vi "Add RUN Window.vi"(6 "Index":i32=-1, 8 "error in (no error)":errorcluster, 9 "Schedule Block":refnum<class "Schedule Block.lvclass">, 10 "Modify":bool, 11 "Scheduler in":refnum<class "Scheduler.lvclass">=refnum) -> (0 "error out":errorcluster={"status"=TRUE, "code"=5666, "source"="desktop-pk571s1: Scheduler: Scheduler::Error while updating subpanels in the Add Run"}, 3 "Scheduler out":refnum<class "Scheduler.lvclass">)   [LabVIEW 2020, in "CIRCUS_uServices.lvlib" / "Scheduler.lvlib"]
uses:
  Scheduler.lvlib
  Run Utilities/Scan SBlock/Scan Mode Panel.vi
  Run Utilities/Scan SBlock/Scan SBlock.lvclass
  Scheduler Consumer Case Selector.ctl
  Scheduler.lvclass
  Add RUN Output Data Packet.ctl
  TALOS/TALOS_PPL.lvlibp
  TALOS/TALOS_PPL.lvlibp/Father of all uServices/Father of all uServices/Father of all uServices.lvclass
  TALOS/TALOS_PPL.lvlibp/Support VIs/Global Memory.vi
  TALOS/TALOS_PPL.lvlibp/Interfaces/FPGA Interface/FPGA Interface.lvclass
  Run Utilities/Schedule Block/Schedule Block.lvclass
  C:/Users/marco/Documents/GitHub_Lab/CIRCUS/TALOS/TALOS_PPL.lvlibp/Father of all uServices/Father of all uServices/Father of all uServices.lvclass
  C:/Users/marco/Documents/GitHub_Lab/CIRCUS/TALOS/TALOS_PPL.lvlibp/Ancestor/Ancestor/Ancestor.lvclass
  C:/Users/marco/Documents/GitHub_Lab/CIRCUS/TALOS/Actor Framework.lvlibp/1abvi3w/vi.lib/ActorFramework/Actor/Actor.lvclass
  C:/Users/marco/Documents/GitHub_Lab/CIRCUS/CIRCUS uServices et al/Scheduler/Scheduler.lvclass
  Run Utilities/Scan SBlock/Parameter name with value - GUI.ctl
  TALOS/Actor Framework.lvlibp/1abvi3w/vi.lib/ActorFramework/Message Enqueuer/Message Enqueuer.lvclass
  TALOS/Actor Framework.lvlibp/1abvi3w/vi.lib/ActorFramework/Message Priority Queue/Message Priority Queue.lvclass
  Classes/Log/Log.lvclass
  Classes/Config/Config.lvclass
panel:
  in  "Subpanels Map":map{string, refnum<vi>}(c390)={"Optimiser"=refnum, "Scan"=refnum}
  in  "Parameters Map":map{string, string[]}(c390)
  in  "FPGA Selector":string(combo)
  in  "Obsv to check":string[](array[string]) caption="Quality of Run Check"
  in  "Mode":string(combo)="Scan"
  in  "Common Parameters":T1[](array[typedef])
  in  "Cancel":bool
  in  "OK":bool
  in  "Number of repetitions":u16=1 min=1
  in  "Browse":bool
  in  "Script Path":path
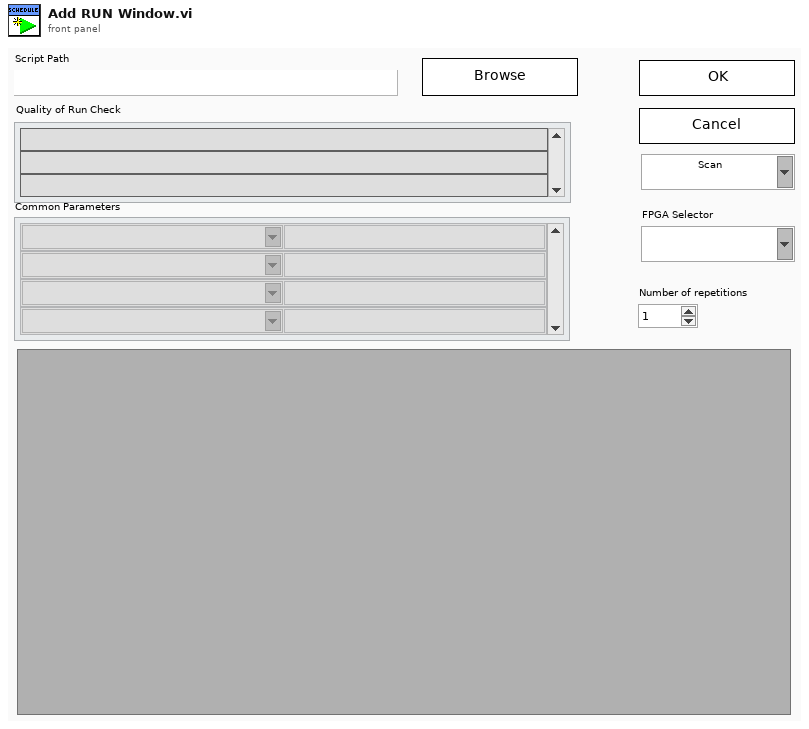
[diagram p1: front panel]
types:
  T1 = typedef "CIRCUS_uServices.lvlib/Run Utilities.lvlib/Scan SBlock.lvclass/Parameter name with value - GUI.ctl" = cluster{"Parameter Name":string, "Parameter Value":string}
  T2 = typedef "CIRCUS_uServices.lvlib/Scheduler.lvlib/Scheduler.lvclass/Add RUN Output Data Packet.ctl" = cluster{"Index":i32, "Schedule Block":refnum<class "Schedule Block.lvclass">}
  T3 = typedef "CIRCUS_uServices.lvlib/Scheduler.lvlib/Scheduler.lvclass/Scheduler Consumer Case Selector.ctl" = enum16{"Add SBlock", "Update GUI", "Move SBlock", "Select SBlock", "Update Cont.", "Load", "Save", "Reset", "Send to Tamer", "Edit SBlock", "Duplicate SBlock", "Delete SBlock", "Update SBlock", "Init", "Split/Combine Schedules", "Reschedule", "Load Parameters"}
  T4 = cluster{"result string":string, "String":string, "result string":string}[]
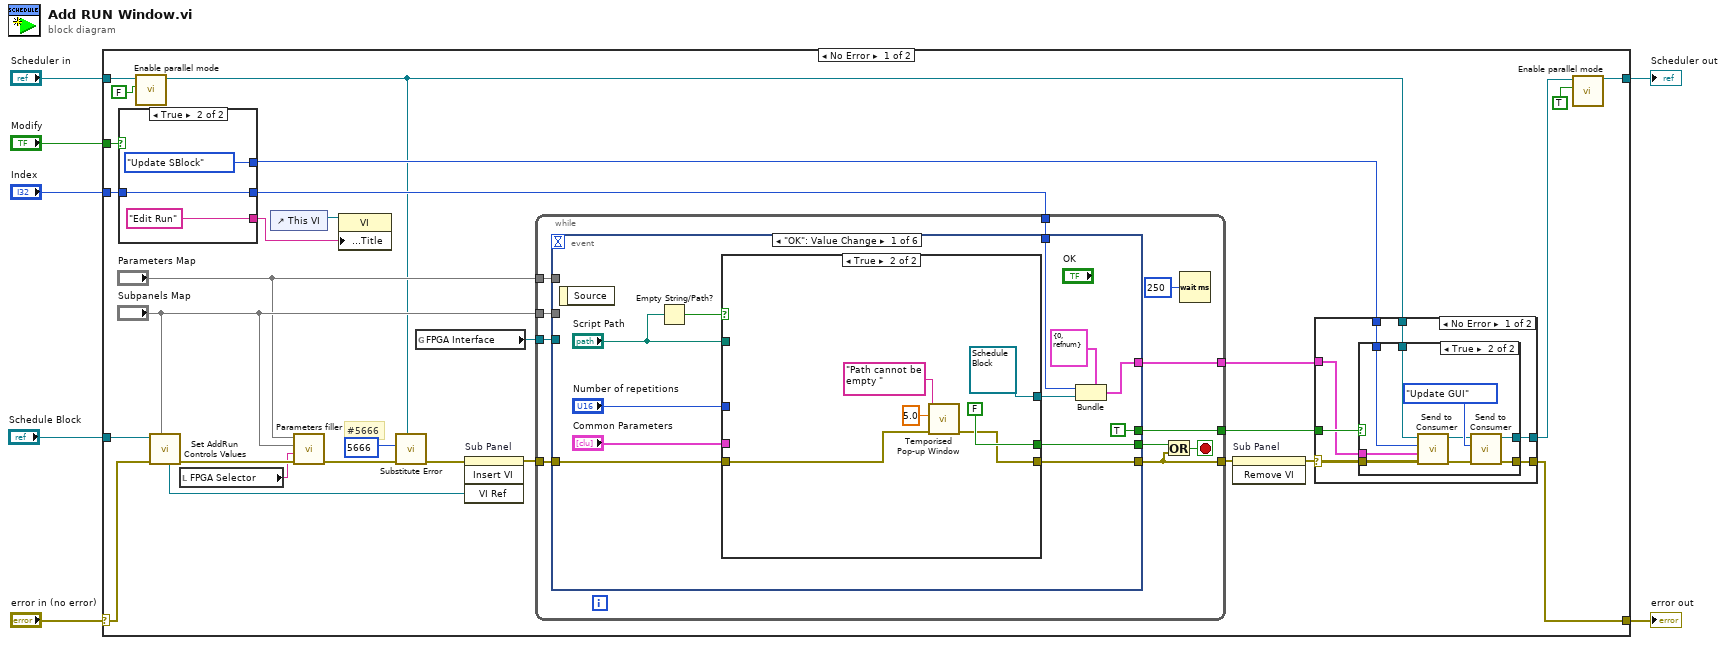
[diagram p0: block diagram]
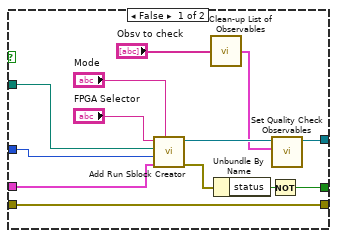
[diagram p2: hidden frame]
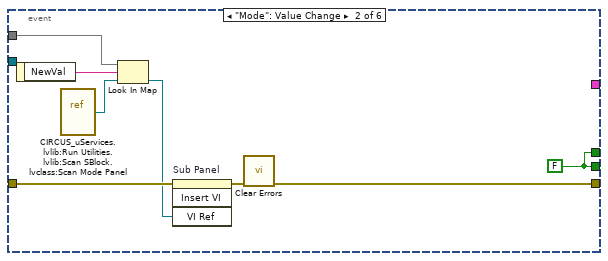
[diagram p3: hidden frame]
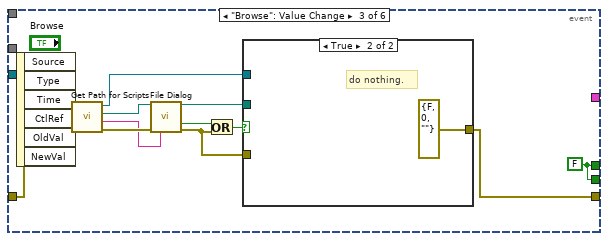
[diagram p4: hidden frame]
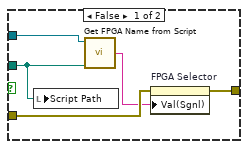
[diagram p5: hidden frame]
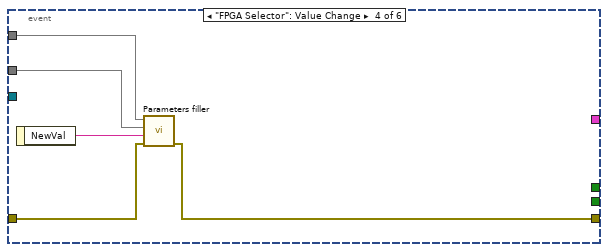
[diagram p6: hidden frame]
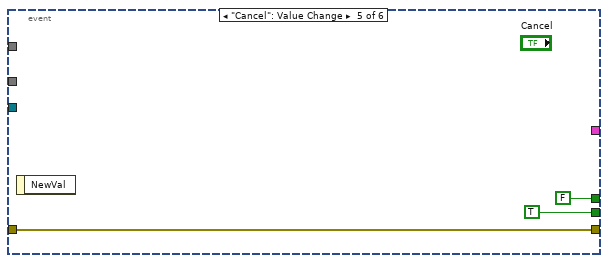
[diagram p7: hidden frame]
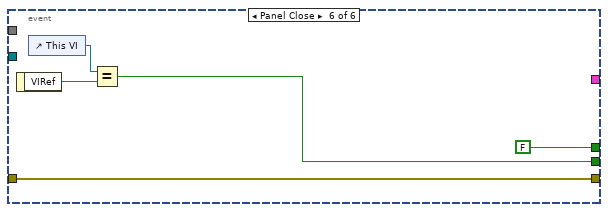
[diagram p8: hidden frame]
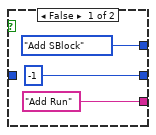
[diagram p11: hidden frame]
diagram:
  n1 = case shown="No Error" "error in (no error)" {
    selector: "error in (no error)" -> [w13 w145]
    tunnel: [w23 w145] -> w4
    tunnel: [w22 w144] -> w5
    tunnel: "Scheduler in" -> [w28 w144]
    tunnel: "Modify" -> [w34 _]
    tunnel: "Schedule Block" -> [w15 _]
    tunnel: "Index" -> [w30 _]
    frame No Error {
      # "#5666"
      n2 = case shown="True" w34 {
        tunnel: [Scheduler_Consumer_Case_Selector."Add SBlock" ("Shifter Panel Consumer Case Selector") Scheduler_Consumer_Case_Selector."Update SBlock" ("Shifter Panel Consumer Case Selector")] -> w32
        tunnel: w30 -> [_ w142]
        tunnel: [-1 ("Index") w142] -> w29
        tunnel: ["Add Run" ("Front Panel Window:Title") "Edit Run" ("Front Panel Window:Title")] -> w19
        frame False {
        }
        frame True {
        }
      }
      n3 = call-dynamic "Enable parallel mode.vi"("Enable"=FALSE, "Scheduler in"=w28) -> ("Scheduler out"=w10:refnum<class "Scheduler.lvclass">)  [unwired: 8 in, 1 out]
      n4 = call "Set AddRun Controls Values.vi"("Subpanels Map"="Subpanels Map", "error in"=w13, "Schedule Block"=w15) -> ("error out"=w16:errorcluster, "SubPanel VI out"=w9:refnum<vi>)  [unwired: 6 in, 1 out]
      n5 = local read "FPGA Selector"() -> (w11:string)
      n6 = control-ref of="This VI"() -> (w18:refnum<vi>)
      n7 = call "Parameters filler.vi"("error in (no error)"=w16, "FPGA Name"=w11, "Subpanels Map"="Subpanels Map", "Parameters Map"="Parameters Map") -> ("error out"=w12:errorcluster)  [unwired: 7 in]
      n8 = property class="VI"(reference=w18, "Front Panel.Title"=w19) -> ()  [unwired: 1 in, 2 out]
      n9 = call "Substitute Error.vi"("LabVIEW Object"=w10, "error in (no error)"=w12, "Error Code"=5666) -> ("error out"=w26:errorcluster)  [unwired: 8 in]
      n10 = global read "Global Memory.vi" "FPGA Interface"() -> (w20:refnum<class "FPGA Interface.lvclass">)
      n11 = invoke on="Sub Panel" class="SubPnl" method="Insert VI"(error in=w26, "VI Ref"=w9) -> (error out=w8:errorcluster)  [unwired: 2 in, 3 out]
      n12 = while {
        tunnel: [w37] -> w35
        tunnel: w8 -> [w47]
        tunnel: [w44] -> w33
        tunnel: [w43] -> w31
        tunnel: w29 -> [w42]
        tunnel: w20 -> [w41]
        tunnel: "Subpanels Map" -> [w40]
        tunnel: "Parameters Map" -> [w39]
        stop <- w46 stop-if-true
        n13 = event shown="[0] \"OK\": Value Change" {
          selector: _ -> [_ _ _ _ _ _]
          dyn-events: _ -> [_ _ _ _ _ _]
          timeout: _ -> [_ _ _ _ _ _]
          tunnel: [w55 w79 w97 _ TRUE w114] -> w38
          tunnel: [w48 w81 w98 w105 w111 w117] -> w37
          tunnel: w47 -> [w56 w82 w91 w106 w111 w117]
          tunnel: [w52 _ _ _ _ _] -> w44
          tunnel: [TRUE w79 w97 _ FALSE FALSE] -> w43
          tunnel: w42 -> [w50 _ _ _ _ _]
          tunnel: w41 -> [_ _ w92 _ _ _]
          tunnel: w40 -> [_ w83 _ w107 _ _]
          tunnel: w39 -> [_ _ _ w108 _ _]
          event "OK": Value Change {
            n14 = event-data() -> ()  [unwired: 1 in, 1 out]
            n15 = Empty String/Path?(string/path="Script Path") -> (empty?=w57:bool)
            n16 = case shown="True" w57 {
              tunnel: "Number of repetitions" -> [w63 _]
              tunnel: "Script Path" -> [w67 _]
              tunnel: w56 -> [w70 w78]
              tunnel: [w72 FALSE] -> w55
              tunnel: [w69 refnum<class "Schedule Block.lvclass"> refnum ("Schedule Block out")] -> w51
              tunnel: "Common Parameters" -> [w66 _]
              tunnel: [w70 w73] -> w48
              frame False {
                n17 = call "Add Run Sblock Creator.vi"("SBlock type"="Mode", "Common Parameters"=w66, "Number of repetitions"=w63, "Script Path"=w67, "FPGA Name"="FPGA Selector") -> ("error out"=w65:errorcluster, "Schedule Block out"=w64:refnum<class "Schedule Block.lvclass">)  [unwired: 5 in]
                n18 = call "Clean-up List of Observables.vi"("Obsv to check"="Obsv to check") -> ("Array"=w60:T4)
                n19 = Unbundle By Name(w65) -> ("status"=w71:bool)
                n20 = Not(x=w71) -> (.not. x?=w72:bool)
                n21 = call-dynamic "Set Quality Check Observables.vi"("Obsv to check"=w60, "Schedule Block in"=w64) -> ("Schedule Block out"=w69:refnum<class "Schedule Block.lvclass">)  [unwired: 8 in, 1 out]
              }
              frame True {
                n22 = call "Temporised Pop-up Window.vi"("error in (no error)"=w78, "Timeout"=5.0, "Text"="Path cannot be empty ") -> ("error out"=w73:errorcluster)  [unwired: 8 in]
              }
            }
            n23 = Bundle(cluster=T2 {"Index"=0, "Schedule Block"=refnum} ("Cluster"), "Index"=w50, "Schedule Block"=w51) -> (w52:T2)
          }
          event "Mode": Value Change {
            w79 = FALSE
            n24 = event-data() -> ("NewVal"=w85:string)  [unwired: 1 in]
            n25 = vi-ref "CIRCUS_uServices.lvlib:Run Utilities.lvlib:Scan SBlock.lvclass:Scan Mode Panel.vi"() -> (w84:refnum<vi>)
            n26 = Look In Map(map=w83, key=w85, default value=w84) -> (value=w80:refnum<vi>)  [unwired: 1 out]
            n27 = invoke on="Sub Panel" class="SubPnl" method="Insert VI"(error in=w82, "VI Ref"=w80) -> (error out=w86:errorcluster)  [unwired: 2 in, 3 out]
            n28 = call <vilib>:"Clear Errors.vi"("error in (no error)"=w86) -> ("error out"=w81:errorcluster)  [unwired: 5 in, 1 out]
          }
          event "Browse": Value Change {
            w97 = FALSE
            n29 = event-data() -> ()  [unwired: 1 in, 6 out]
            n30 = call-dynamic "Get Path for Scripts.vi"("error in (no error)"=w91, "FPGA Interface in"=w92) -> ("error out"=w90:errorcluster, "File pattern"=w89:string, "Path"=w88:path, "FPGA Interface out"=w87:refnum<class "FPGA Interface.lvclass">)  [unwired: 6 in]
            n31 = call "File Dialog"("start path"=w88, "error in"=w90, "pattern (all files)"=w89) -> ("selected path"=w94:path, "cancelled"=w96:bool, "error out"=w93:errorcluster)  [unwired: 9 in, 1 out]
            n32 = Or(x=w96, y=w93) -> (x .or. y?=w95:bool)
            n33 = case shown="True" w95 {
              tunnel: w94 -> [w103 _]
              tunnel: [w101 errorcluster {"status"=FALSE, "code"=0, "source"=""} ("error out")] -> w98
              tunnel: w93 -> [w100 _]
              tunnel: w87 -> [w102 _]
              frame False {
                n34 = local write "Script Path"(w103) -> ()
                n35 = call-dynamic "Get FPGA Name from Script.vi"("file"=w103, "FPGA Interface"=w102) -> ("FPGA Name"=w99:string)  [unwired: 2 in]
                n36 = property on="FPGA Selector" class="CmbBox"(error in=w100, "Val(Sgnl)"=w99) -> (error out=w101:errorcluster)  [unwired: 1 in, 1 out]
              }
              frame True {
                # "do nothing."
              }
            }
          }
          event "FPGA Selector": Value Change {
            n37 = event-data() -> ("NewVal"=w109:string)  [unwired: 1 in]
            n38 = call "Parameters filler.vi"("error in (no error)"=w106, "FPGA Name"=w109, "Subpanels Map"=w107, "Parameters Map"=w108) -> ("error out"=w105:errorcluster)  [unwired: 7 in]
          }
          event "Cancel": Value Change {
            n39 = event-data() -> ()  [unwired: 1 in, 1 out]
          }
          event Panel Close {
            n40 = event-data() -> ("VIRef"=w116:refnum<vi>)  [unwired: 1 in]
            n41 = control-ref of="This VI"() -> (w115:refnum<vi>)
            n42 = Equal?(x=w115, y=w116) -> (x = y?=w114:bool)
          }
        }
        n43 = Or(x=w38, y=w37) -> (x .or. y?=w46:bool)
        n44 = Wait (ms)(milliseconds to wait=u32 250) -> ()  [unwired: 1 out]
      }
      n45 = invoke on="Sub Panel" class="SubPnl" method="Remove VI"(error in=w35) -> (error out=w36:errorcluster)  [unwired: 2 in, 2 out]
      n46 = case shown="No Error" w36 {
        selector: w36 -> [w124 w137]
        tunnel: [w123 w137] -> w23
        tunnel: w33 -> [w119 _]
        tunnel: w10 -> [w122 w136]
        tunnel: w32 -> [w121 _]
        tunnel: w31 -> [w120 _]
        tunnel: [w118 w136] -> w24
        frame No Error {
          n47 = case shown="True" w120 {
            tunnel: w124 -> [w126 w135]
            tunnel: [w126 w129] -> w123
            tunnel: w119 -> [_ w134]
            tunnel: w122 -> [w125 w133]
            tunnel: w121 -> [_ w132]
            tunnel: [w125 w128] -> w118
            frame False {
            }
            frame True {
              n48 = call "Send to Consumer.vi"("error in (no error)"=w135, "Data"=w134, "Case ID"=w132, "uService Template in"=w133) -> ("error out"=w131:errorcluster, "uService Template out"=w127:refnum<class "Scheduler.lvclass">)  [unwired: 6 in]
              n49 = call "Send to Consumer.vi"("error in (no error)"=w131, "Case ID"=Scheduler_Consumer_Case_Selector."Update GUI" ("Consumer Case Selector"), "uService Template in"=w127) -> ("error out"=w129:errorcluster, "uService Template out"=w128:refnum<class "Scheduler.lvclass">)  [unwired: 7 in]
            }
          }
        }
        frame Error {
        }
      }
      n50 = call-dynamic "Enable parallel mode.vi"("Enable"=TRUE, "Scheduler in"=w24) -> ("Scheduler out"=w22:refnum<class "Scheduler.lvclass">)  [unwired: 8 in, 1 out]
    }
    frame Error {
    }
  }
  "error out" <- w4
  "Scheduler out" <- w5
